vi "stop.vi"(8 "error in (no error)":errorcluster, 10 "stop?":bool, 11 "AtomChipHWC in":refnum<class "AtomChipHWC.lvclass">) -> (0 "error out":errorcluster, 2 "stopped":bool, 3 "AtomChipHWC out":refnum<class "AtomChipHWC.lvclass">)   [LabVIEW 2011, in "Hardware.lvlib" / "HWControllers.lvlib" / "AtomChipHWC.lvclass"]
doc: "Stop current run if input is true, otherwise ask hardware if its finished."
uses:
  AtomChipHWC.lvclass
  AtomChipHWC.lvclass/AtomChipHWC.ctl
  Channels/Digital/DigitalOutput.lvclass
  Channels/VoltOutput/AnalogOutput.lvclass
  Channels/DDSOutput/Generic/DDSOutput.lvclass
  Network Controllers/NetworkCamera/NetworkCamera.lvclass
  IntegrationManagement/CameraManager.lvclass
  HWController.lvclass
  Network Controllers/CameraNetworkController/CameraNetworkController.lvclass
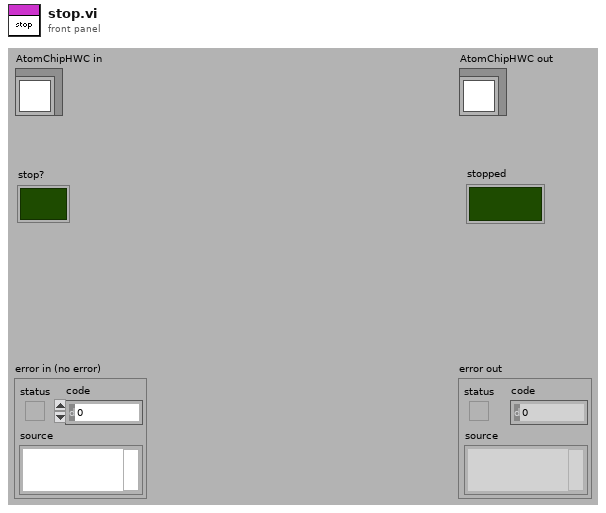
[diagram p1: front panel]
types:
  T1 = enum16{"Ready", "Compiling", "Configured", "Running", "Stopping", "Unresolved Error"}
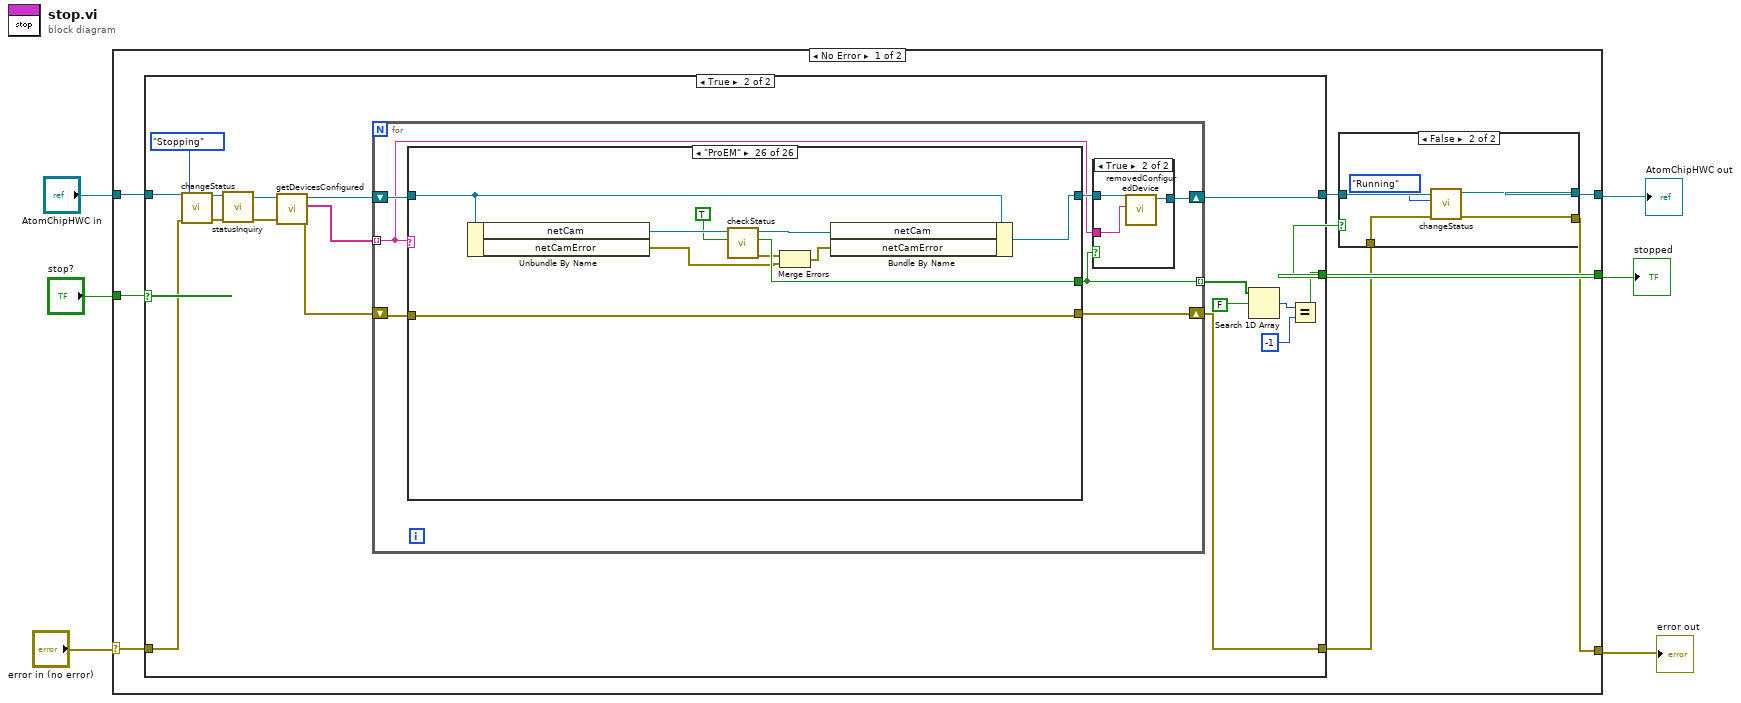
[diagram p0: block diagram]
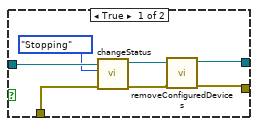
[diagram p2: hidden frame]
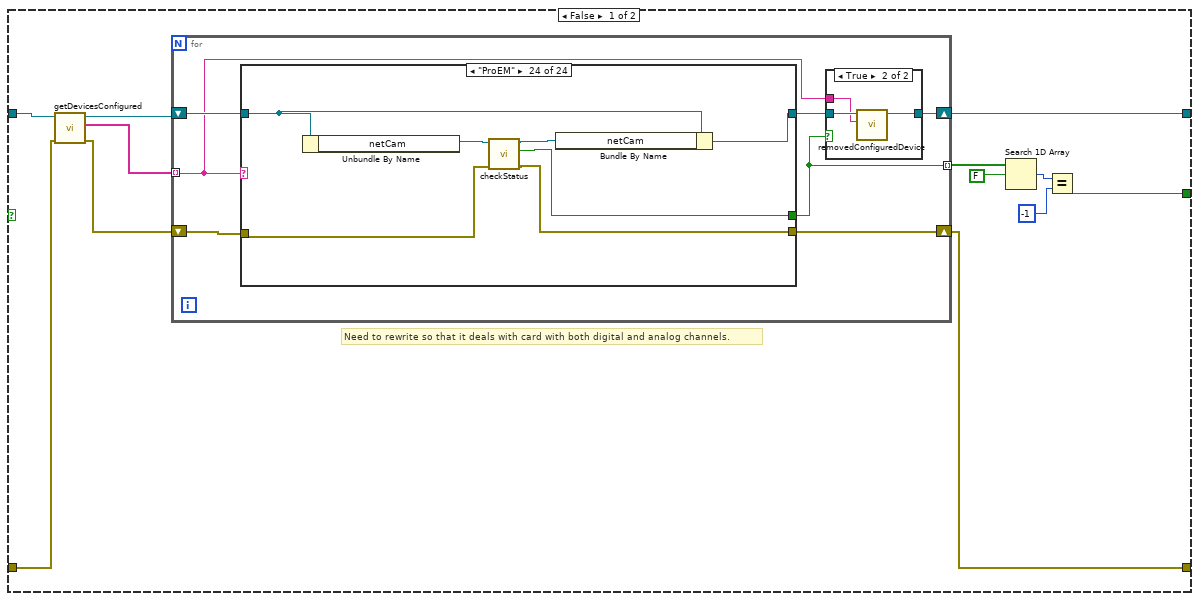
[diagram p3: hidden frame]
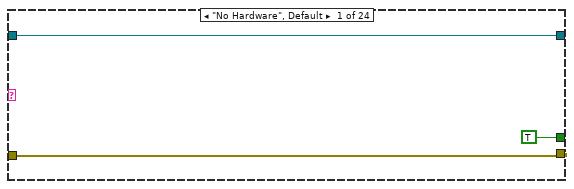
[diagram p5: hidden frame]
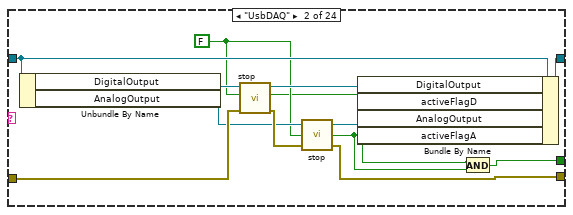
[diagram p6: hidden frame]
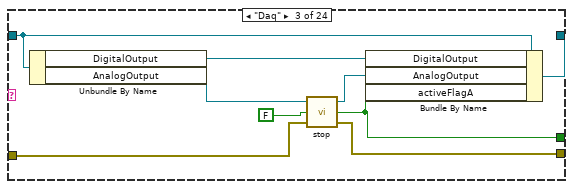
[diagram p7: hidden frame]
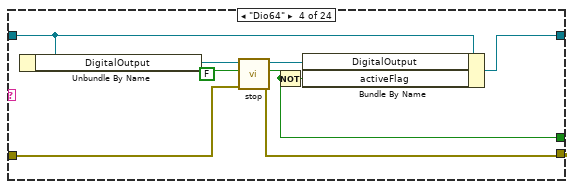
[diagram p8: hidden frame]
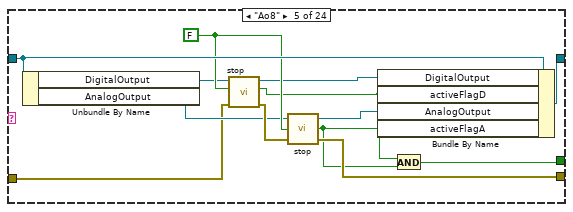
[diagram p9: hidden frame]
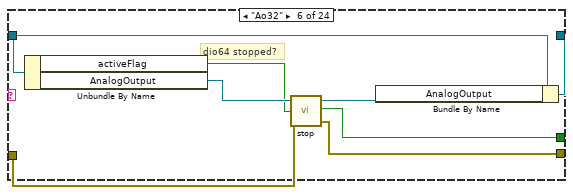
[diagram p10: hidden frame]
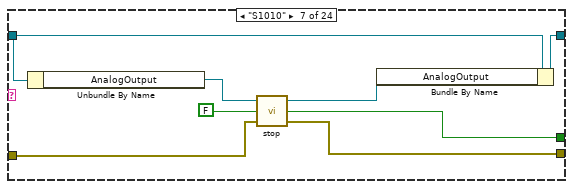
[diagram p11: hidden frame]
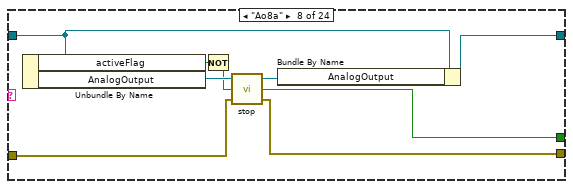
[diagram p12: hidden frame]
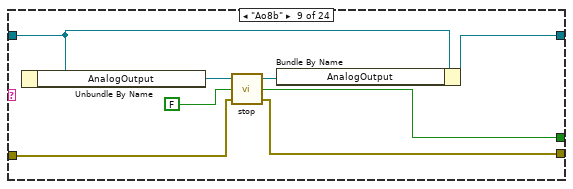
[diagram p13: hidden frame]
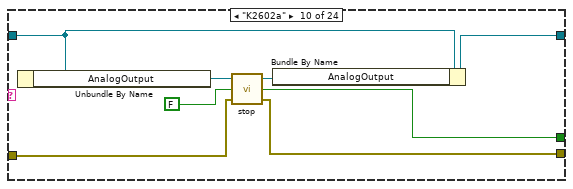
[diagram p14: hidden frame]
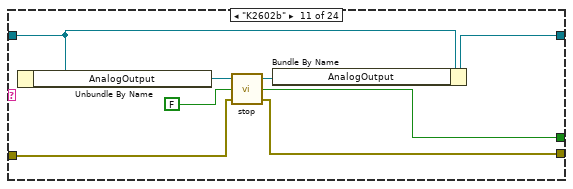
[diagram p15: hidden frame]
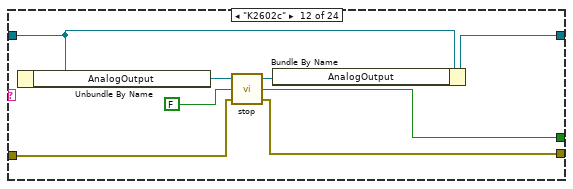
[diagram p16: hidden frame]
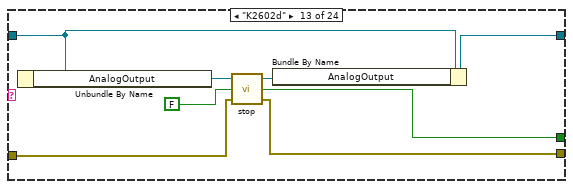
[diagram p17: hidden frame]
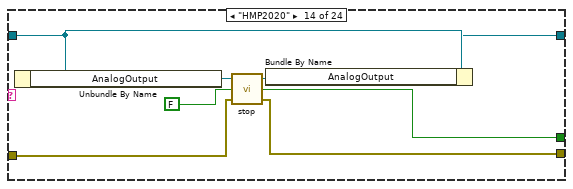
[diagram p18: hidden frame]
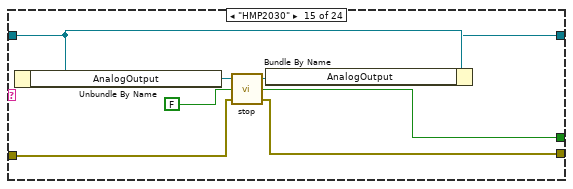
[diagram p19: hidden frame]
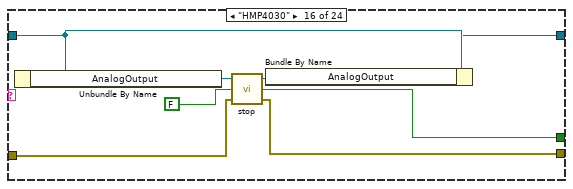
[diagram p20: hidden frame]
diagram:
  n1 = case shown="No Error" "error in (no error)" {
    selector: "error in (no error)" -> [w13 w549]
    tunnel: "AtomChipHWC in" -> [w14 w550]
    tunnel: [w8 w550] -> w5
    tunnel: [w7 w549] -> w3
    tunnel: "stop?" -> [w12 _]
    tunnel: [w9 _] -> w1
    frame No Error {
      n2 = case shown="True" w12 {
        tunnel: w14 -> [w31 w263]
        tunnel: [w38 w261] -> w11
        tunnel: w13 -> [w29 w262]
        tunnel: [w37 w260] -> w10
        tunnel: [w32 w247] -> w9
        frame False {
          # "Need to rewrite so that it deals with card with both digital and analog channels."
          n3 = call "getDevicesConfigured.vi"("error in (no error)"=w29, "HWController.lvclass in"=w31) -> ("error out"=w28:errorcluster, "devicesConfigured"=w27:string[], "HWController.lvclass out"=w30:refnum<class "AtomChipHWC.lvclass">)  [unwired: 7 in]
          n4 = for {
            shift-right: [w40] -> w38
            shift-left: w30 -> [w45]
            tunnel: w27 -> [w41] mode=indexing
            shift-right: [w44] -> w37
            shift-left: w28 -> [w43]
            tunnel: [w42] -> w36 mode=indexing
            n5 = case shown="\"ProEM\"" w41 {
              tunnel: [w52 w64 w74 w79 w95 w104 w112 w115 w123 w131 w139 w147 w155 w163 w171 w179 w186 w194 w203 w212 w222 w231 w238 w245] -> w39
              tunnel: [w51 w61 w69 w81 w88 w101 w109 w119 w127 w135 w143 w151 w159 w167 w175 w183 w190 w198 w207 w216 w220 w227 w234 w241] -> w44
              tunnel: w45 -> [w52 w65 w72 w78 w96 w103 w111 w117 w125 w133 w141 w149 w157 w165 w173 w181 w188 w196 w205 w214 w223 w232 w239 w246]
              tunnel: w43 -> [w51 w59 w66 w82 w89 w99 w107 w120 w128 w136 w144 w152 w160 w168 w176 w184 w191 w199 w208 w217 w224 w228 w235 w242]
              tunnel: [TRUE w53 w67 w76 w84 w98 w105 w118 w126 w134 w142 w150 w158 w166 w174 w182 w189 w197 w206 w215 w221 w226 w233 w240] -> w42
              frame "No Hardware", Default {
              }
              frame "UsbDAQ" {
                w57 = FALSE
                n6 = Unbundle By Name(w65) -> ("DigitalOutput"=w63:refnum<class "DigitalOutput.lvclass">, "AnalogOutput"=w58:refnum<class "AnalogOutput.lvclass">)
                n7 = call-dynamic "stop.vi"("error in (no error)"=w59, "stop"=w57, "DigitalOutput in"=w63) -> ("error out"=w60:errorcluster, "stopped"=w54:bool, "DigitalOutput out"=w62:refnum<class "DigitalOutput.lvclass">)  [unwired: 6 in]
                n8 = call-dynamic "stop.vi"("error in (no error)"=w60, "stop"=w57, "AnalogOutput in"=w58) -> ("error out"=w61:errorcluster, "Stopped"=w55:bool, "AnalogOutput out"=w56:refnum<class "AnalogOutput.lvclass">)
                n9 = Bundle By Name(cluster=w65, "DigitalOutput"=w62, "activeFlagD"=w54, "AnalogOutput"=w56, "activeFlagA"=w55) -> (w64:refnum<class "AtomChipHWC.lvclass">)
                n10 = And(x=w54, y=w55) -> (x .and. y?=w53:bool)
              }
              frame "Daq" {
                n11 = Unbundle By Name(w72) -> ("DigitalOutput"=w68:refnum<class "DigitalOutput.lvclass">, "AnalogOutput"=w71:refnum<class "AnalogOutput.lvclass">)
                n12 = call-dynamic "stop.vi"("error in (no error)"=w66, "stop"=FALSE, "AnalogOutput in"=w71) -> ("error out"=w69:errorcluster, "Stopped"=w67:bool, "AnalogOutput out"=w70:refnum<class "AnalogOutput.lvclass">)
                n13 = Bundle By Name(cluster=w72, "DigitalOutput"=w68, "AnalogOutput"=w70, "activeFlagA"=w67) -> (w74:refnum<class "AtomChipHWC.lvclass">)
              }
              frame "Dio64" {
                n14 = Unbundle By Name(w78) -> ("DigitalOutput"=w83:refnum<class "DigitalOutput.lvclass">)
                n15 = call-dynamic "stop.vi"("error in (no error)"=w82, "stop"=FALSE, "DigitalOutput in"=w83) -> ("error out"=w81:errorcluster, "stopped"=w76:bool, "DigitalOutput out"=w80:refnum<class "DigitalOutput.lvclass">)  [unwired: 6 in]
                n16 = Not(x=w76) -> (.not. x?=w75:bool)
                n17 = Bundle By Name(cluster=w78, "DigitalOutput"=w80, "activeFlag"=w75) -> (w79:refnum<class "AtomChipHWC.lvclass">)
              }
              frame "Ao8" {
                w93 = FALSE
                n18 = Unbundle By Name(w96) -> ("DigitalOutput"=w92:refnum<class "DigitalOutput.lvclass">, "AnalogOutput"=w91:refnum<class "AnalogOutput.lvclass">)
                n19 = call-dynamic "stop.vi"("error in (no error)"=w89, "stop"=w93, "DigitalOutput in"=w92) -> ("error out"=w94:errorcluster, "stopped"=w86:bool, "DigitalOutput out"=w90:refnum<class "DigitalOutput.lvclass">)  [unwired: 6 in]
                n20 = call-dynamic "stop.vi"("error in (no error)"=w94, "stop"=w93, "AnalogOutput in"=w91) -> ("error out"=w88:errorcluster, "Stopped"=w85:bool, "AnalogOutput out"=w87:refnum<class "AnalogOutput.lvclass">)
                n21 = Bundle By Name(cluster=w96, "DigitalOutput"=w90, "activeFlagD"=w86, "AnalogOutput"=w87, "activeFlagA"=w85) -> (w95:refnum<class "AtomChipHWC.lvclass">)
                n22 = And(x=w86, y=w85) -> (x .and. y?=w84:bool)
              }
              frame "Ao32" {
                # "dio64 stopped?"
                n23 = Unbundle By Name(w103) -> ("activeFlag"=w97:bool, "AnalogOutput"=w102:refnum<class "AnalogOutput.lvclass">)
                n24 = call-dynamic "stop.vi"("error in (no error)"=w99, "stop"=w97, "AnalogOutput in"=w102) -> ("error out"=w101:errorcluster, "Stopped"=w98:bool, "AnalogOutput out"=w100:refnum<class "AnalogOutput.lvclass">)
                n25 = Bundle By Name(cluster=w103, "AnalogOutput"=w100) -> (w104:refnum<class "AtomChipHWC.lvclass">)
              }
              frame "S1010" {
                n26 = Unbundle By Name(w111) -> ("AnalogOutput"=w110:refnum<class "AnalogOutput.lvclass">)
                n27 = call-dynamic "stop.vi"("error in (no error)"=w107, "stop"=FALSE, "AnalogOutput in"=w110) -> ("error out"=w109:errorcluster, "Stopped"=w105:bool, "AnalogOutput out"=w108:refnum<class "AnalogOutput.lvclass">)
                n28 = Bundle By Name(cluster=w111, "AnalogOutput"=w108) -> (w112:refnum<class "AtomChipHWC.lvclass">)
              }
              frame "Ao8a" {
                n29 = Unbundle By Name(w117) -> ("activeFlag"=w114:bool, "AnalogOutput"=w121:refnum<class "AnalogOutput.lvclass">)
                n30 = Not(x=w114) -> (.not. x?=w113:bool)
                n31 = call-dynamic "stop.vi"("error in (no error)"=w120, "stop"=w113, "AnalogOutput in"=w121) -> ("error out"=w119:errorcluster, "Stopped"=w118:bool, "AnalogOutput out"=w116:refnum<class "AnalogOutput.lvclass">)
                n32 = Bundle By Name(cluster=w117, "AnalogOutput"=w116) -> (w115:refnum<class "AtomChipHWC.lvclass">)
              }
              frame "Ao8b" {
                n33 = Unbundle By Name(w125) -> ("AnalogOutput"=w129:refnum<class "AnalogOutput.lvclass">)
                n34 = call-dynamic "stop.vi"("error in (no error)"=w128, "stop"=FALSE, "AnalogOutput in"=w129) -> ("error out"=w127:errorcluster, "Stopped"=w126:bool, "AnalogOutput out"=w124:refnum<class "AnalogOutput.lvclass">)
                n35 = Bundle By Name(cluster=w125, "AnalogOutput"=w124) -> (w123:refnum<class "AtomChipHWC.lvclass">)
              }
              frame "K2602a" {
                n36 = Unbundle By Name(w133) -> ("AnalogOutput"=w137:refnum<class "AnalogOutput.lvclass">)
                n37 = call-dynamic "stop.vi"("error in (no error)"=w136, "stop"=FALSE, "AnalogOutput in"=w137) -> ("error out"=w135:errorcluster, "Stopped"=w134:bool, "AnalogOutput out"=w132:refnum<class "AnalogOutput.lvclass">)
                n38 = Bundle By Name(cluster=w133, "AnalogOutput"=w132) -> (w131:refnum<class "AtomChipHWC.lvclass">)
              }
              frame "K2602b" {
                n39 = Unbundle By Name(w141) -> ("AnalogOutput"=w145:refnum<class "AnalogOutput.lvclass">)
                n40 = call-dynamic "stop.vi"("error in (no error)"=w144, "stop"=FALSE, "AnalogOutput in"=w145) -> ("error out"=w143:errorcluster, "Stopped"=w142:bool, "AnalogOutput out"=w140:refnum<class "AnalogOutput.lvclass">)
                n41 = Bundle By Name(cluster=w141, "AnalogOutput"=w140) -> (w139:refnum<class "AtomChipHWC.lvclass">)
              }
              frame "K2602c" {
                n42 = Unbundle By Name(w149) -> ("AnalogOutput"=w153:refnum<class "AnalogOutput.lvclass">)
                n43 = call-dynamic "stop.vi"("error in (no error)"=w152, "stop"=FALSE, "AnalogOutput in"=w153) -> ("error out"=w151:errorcluster, "Stopped"=w150:bool, "AnalogOutput out"=w148:refnum<class "AnalogOutput.lvclass">)
                n44 = Bundle By Name(cluster=w149, "AnalogOutput"=w148) -> (w147:refnum<class "AtomChipHWC.lvclass">)
              }
              frame "K2602d" {
                n45 = Unbundle By Name(w157) -> ("AnalogOutput"=w161:refnum<class "AnalogOutput.lvclass">)
                n46 = call-dynamic "stop.vi"("error in (no error)"=w160, "stop"=FALSE, "AnalogOutput in"=w161) -> ("error out"=w159:errorcluster, "Stopped"=w158:bool, "AnalogOutput out"=w156:refnum<class "AnalogOutput.lvclass">)
                n47 = Bundle By Name(cluster=w157, "AnalogOutput"=w156) -> (w155:refnum<class "AtomChipHWC.lvclass">)
              }
              frame "HMP2020" {
                n48 = Unbundle By Name(w165) -> ("AnalogOutput"=w169:refnum<class "AnalogOutput.lvclass">)
                n49 = call-dynamic "stop.vi"("error in (no error)"=w168, "stop"=FALSE, "AnalogOutput in"=w169) -> ("error out"=w167:errorcluster, "Stopped"=w166:bool, "AnalogOutput out"=w164:refnum<class "AnalogOutput.lvclass">)
                n50 = Bundle By Name(cluster=w165, "AnalogOutput"=w164) -> (w163:refnum<class "AtomChipHWC.lvclass">)
              }
              frame "HMP2030" {
                n51 = Unbundle By Name(w173) -> ("AnalogOutput"=w177:refnum<class "AnalogOutput.lvclass">)
                n52 = call-dynamic "stop.vi"("error in (no error)"=w176, "stop"=FALSE, "AnalogOutput in"=w177) -> ("error out"=w175:errorcluster, "Stopped"=w174:bool, "AnalogOutput out"=w172:refnum<class "AnalogOutput.lvclass">)
                n53 = Bundle By Name(cluster=w173, "AnalogOutput"=w172) -> (w171:refnum<class "AtomChipHWC.lvclass">)
              }
              frame "HMP4030" {
                n54 = Unbundle By Name(w181) -> ("AnalogOutput"=w185:refnum<class "AnalogOutput.lvclass">)
                n55 = call-dynamic "stop.vi"("error in (no error)"=w184, "stop"=FALSE, "AnalogOutput in"=w185) -> ("error out"=w183:errorcluster, "Stopped"=w182:bool, "AnalogOutput out"=w180:refnum<class "AnalogOutput.lvclass">)
                n56 = Bundle By Name(cluster=w181, "AnalogOutput"=w180) -> (w179:refnum<class "AtomChipHWC.lvclass">)
              }
              frame "SpinCoreDDS0" {
                n57 = Unbundle By Name(w188) -> ("DDSOutput"=w192:refnum<class "DDSOutput.lvclass">)
                n58 = call-dynamic "stop.vi"("error in (no error)"=w191, "DDSOutput in"=w192) -> ("error out"=w190:errorcluster, "hasStopped"=w189:bool, "DDSOutput out"=w187:refnum<class "DDSOutput.lvclass">)  [unwired: 7 in]
                n59 = Bundle By Name(cluster=w188, "DDSOutput"=w187) -> (w186:refnum<class "AtomChipHWC.lvclass">)
              }
              frame "SpinCoreDDS1" {
                n60 = Unbundle By Name(w196) -> ("DDSOutput"=w200:refnum<class "DDSOutput.lvclass">)
                n61 = call-dynamic "stop.vi"("error in (no error)"=w199, "stop?"=FALSE, "DDSOutput in"=w200) -> ("error out"=w198:errorcluster, "hasStopped"=w197:bool, "DDSOutput out"=w195:refnum<class "DDSOutput.lvclass">)  [unwired: 6 in]
                n62 = Bundle By Name(cluster=w196, "DDSOutput"=w195) -> (w194:refnum<class "AtomChipHWC.lvclass">)
              }
              frame "k3390" {
                # "stop when Dio64 has stopped."
                n63 = Unbundle By Name(w205) -> ("DDSOutput"=w209:refnum<class "DDSOutput.lvclass">, "activeFlag"=w201:bool)
                n64 = Not(x=w201) -> (.not. x?=w202:bool)
                n65 = call-dynamic "stop.vi"("error in (no error)"=w208, "stop?"=w202, "DDSOutput in"=w209) -> ("error out"=w207:errorcluster, "hasStopped"=w206:bool, "DDSOutput out"=w204:refnum<class "DDSOutput.lvclass">)  [unwired: 6 in]
                n66 = Bundle By Name(cluster=w205, "DDSOutput"=w204) -> (w203:refnum<class "AtomChipHWC.lvclass">)
              }
              frame "CQTDDS0" {
                # "stop when Dio64 has stopped."
                n67 = Unbundle By Name(w214) -> ("DDSOutput"=w218:refnum<class "DDSOutput.lvclass">, "activeFlag"=w211:bool)
                n68 = Not(x=w211) -> (.not. x?=w210:bool)
                n69 = call-dynamic "stop.vi"("error in (no error)"=w217, "stop?"=w210, "DDSOutput in"=w218) -> ("error out"=w216:errorcluster, "hasStopped"=w215:bool, "DDSOutput out"=w213:refnum<class "DDSOutput.lvclass">)  [unwired: 6 in]
                n70 = Bundle By Name(cluster=w214, "DDSOutput"=w213) -> (w212:refnum<class "AtomChipHWC.lvclass">)
              }
              frame "oldPixelfly", "oldProEM_WinX32" {
                n71 = Unbundle By Name(w223) -> ("CameraNetworkController"=w225:refnum<class "CameraNetworkController.lvclass">)
                n72 = call "stop.vi"("error in (no error)"=w224, "CameraNetworkController in"=w225) -> ("error out"=w220:errorcluster, "stopped?"=w221:bool, "CameraNetworkController out"=w219:refnum<class "CameraNetworkController.lvclass">)  [unwired: 7 in]
                n73 = Bundle By Name(cluster=w223, "CameraNetworkController"=w219) -> (w222:refnum<class "AtomChipHWC.lvclass">)
              }
              frame "Pixelfly" {
                n74 = Unbundle By Name(w232) -> ("netCam"=w230:refnum<class "NetworkCamera.lvclass">)
                n75 = call-dynamic "checkStatus.vi"("error in (no error)"=w228, "NetworkCamera in"=w230) -> ("error out"=w227:errorcluster, "stopped?"=w226:bool, "NetworkCamera out"=w229:refnum<class "NetworkCamera.lvclass">)  [unwired: 7 in]
                n76 = Bundle By Name(cluster=w232, "netCam"=w229) -> (w231:refnum<class "AtomChipHWC.lvclass">)
              }
              frame "Pixis" {
                n77 = Unbundle By Name(w239) -> ("netCam"=w237:refnum<class "NetworkCamera.lvclass">)
                n78 = call-dynamic "checkStatus.vi"("error in (no error)"=w235, "NetworkCamera in"=w237) -> ("error out"=w234:errorcluster, "stopped?"=w233:bool, "NetworkCamera out"=w236:refnum<class "NetworkCamera.lvclass">)  [unwired: 7 in]
                n79 = Bundle By Name(cluster=w239, "netCam"=w236) -> (w238:refnum<class "AtomChipHWC.lvclass">)
              }
              frame "ProEM" {
                n80 = Unbundle By Name(w246) -> ("netCam"=w244:refnum<class "NetworkCamera.lvclass">)
                n81 = call-dynamic "checkStatus.vi"("error in (no error)"=w242, "NetworkCamera in"=w244) -> ("error out"=w241:errorcluster, "stopped?"=w240:bool, "NetworkCamera out"=w243:refnum<class "NetworkCamera.lvclass">)  [unwired: 7 in]
                n82 = Bundle By Name(cluster=w246, "netCam"=w243) -> (w245:refnum<class "AtomChipHWC.lvclass">)
              }
            }
            n83 = case shown="True" w42 {
              tunnel: w41 -> [_ w47]
              tunnel: [w46 w48] -> w40
              tunnel: w39 -> [w46 w49]
              frame False {
              }
              frame True {
                n84 = call-dynamic "removedConfiguredDevice.vi"("device"=w47, "HWController in"=w49) -> ("HWController out"=w48:refnum<class "AtomChipHWC.lvclass">)  [unwired: 8 in, 1 out]
              }
            }
          }
          n85 = Search 1D Array(1D array=w36, element=FALSE) -> (index of element=w34:i32)  [unwired: 1 in]
          n86 = Equal?(x=w34, y=-1) -> (x = y?=w32:bool)
        }
        frame True {
          n87 = call "changeStatus.vi"("error in (no error)"=w262, "status"=T1."Stopping", "HWController in"=w263) -> ("error out"=w258:errorcluster, "HWController out"=w259:refnum<class "AtomChipHWC.lvclass">)  [unwired: 7 in]
          n88 = call-dynamic "statusInquiry.vi"("error in (no error)"=w258, "HWController in"=w259) -> ("error out"=w254:errorcluster, "HWController out"=w257:refnum<class "AtomChipHWC.lvclass">)  [unwired: 8 in]
          n89 = call "getDevicesConfigured.vi"("error in (no error)"=w254, "HWController.lvclass in"=w257) -> ("error out"=w253:errorcluster, "devicesConfigured"=w255:string[], "HWController.lvclass out"=w256:refnum<class "AtomChipHWC.lvclass">)  [unwired: 7 in]
          n90 = for {
            tunnel: w255 -> [w265] mode=indexing
            shift-right: [w266] -> w261
            shift-left: w256 -> [w270]
            shift-right: [w268] -> w260
            shift-left: w253 -> [w269]
            tunnel: [w264] -> w248 mode=indexing
            n91 = case shown="\"ProEM\"" w265 {
              tunnel: [w277 w284 w317 w325 w342 w369 w375 w383 w391 w399 w408 w417 w426 w435 w444 w453 w462 w471 w482 w491 w500 w509 w519 w528 w537 w547] -> w267
              tunnel: [w276 w278 w310 w320 w329 w361 w370 w381 w387 w395 w404 w413 w422 w431 w440 w449 w458 w467 w476 w485 w494 w503 w514 w527 w536 w546] -> w268
              tunnel: w270 -> [w277 w283 w316 w326 w341 w368 w376 w385 w393 w400 w409 w418 w427 w436 w445 w454 w463 w472 w483 w492 w501 w510 w520 w529 w538 w548]
              tunnel: w269 -> [w276 w278 w310 w320 w329 w361 w370 w381 w387 w395 w404 w413 w422 w431 w440 w449 w458 w467 w476 w485 w494 w503 w514 w527 w536 w546]
              tunnel: [FALSE w282 w313 w324 w334 w364 w374 TRUE TRUE w398 w407 w416 w425 w434 w443 w452 w461 w470 w480 w489 w498 w507 w515 w521 w530 w542] -> w264
              frame "No Hardware", Default {
              }
              frame "UsbDAQ" {
                n92 = Unbundle By Name(w283) -> ("DigitalOutput"=w291:refnum<class "DigitalOutput.lvclass">, "AnalogOutput"=w288:refnum<class "AnalogOutput.lvclass">, "activeFlagD"=w290:bool, "activeFlagA"=w287:bool, "UsbDAQError"=w279:errorcluster)
                n93 = case shown="False" w290 {
                  selector: w290 -> [_ w307]
                  tunnel: w291 -> [w306 w309]
                  tunnel: [w305 w309] -> w289
                  tunnel: w279 -> [w304 w308]
                  tunnel: [w303 w308] -> w281
                  tunnel: [w301 w307] -> w286
                  frame False {
                    n94 = call-dynamic "stop.vi"("error in (no error)"=w304, "stop"=TRUE, "DigitalOutput in"=w306) -> ("error out"=w303:errorcluster, "stopped"=w301:bool, "DigitalOutput out"=w305:refnum<class "DigitalOutput.lvclass">)  [unwired: 6 in]
                  }
                  frame True {
                  }
                }
                n95 = case shown="False" w287 {
                  selector: w287 -> [_ w298]
                  tunnel: w281 -> [w297 w299]
                  tunnel: w288 -> [w296 w300]
                  tunnel: [w294 w300] -> w285
                  tunnel: [w293 w299] -> w280
                  tunnel: [w292 w298] -> w282
                  frame False {
                    n96 = call-dynamic "stop.vi"("error in (no error)"=w297, "stop"=TRUE, "AnalogOutput in"=w296) -> ("error out"=w293:errorcluster, "Stopped"=w292:bool, "AnalogOutput out"=w294:refnum<class "AnalogOutput.lvclass">)
                  }
                  frame True {
                  }
                }
                n97 = Bundle By Name(cluster=w283, "DigitalOutput"=w289, "AnalogOutput"=w285, "activeFlagD"=w286, "activeFlagA"=w282, "UsbDAQError"=w280) -> (w284:refnum<class "AtomChipHWC.lvclass">)
              }
              frame "Daq" {
                n98 = Unbundle By Name(w316) -> ("DigitalOutput"=w315:refnum<class "DigitalOutput.lvclass">, "AnalogOutput"=w319:refnum<class "AnalogOutput.lvclass">, "daqError"=w311:errorcluster)
                n99 = call-dynamic "stop.vi"("error in (no error)"=w311, "stop"=TRUE, "AnalogOutput in"=w319) -> ("error out"=w312:errorcluster, "Stopped"=w313:bool, "AnalogOutput out"=w318:refnum<class "AnalogOutput.lvclass">)
                n100 = Bundle By Name(cluster=w316, "DigitalOutput"=w315, "AnalogOutput"=w318, "activeFlagA"=w313, "daqError"=w312) -> (w317:refnum<class "AtomChipHWC.lvclass">)
              }
              frame "Dio64" {
                n101 = Unbundle By Name(w326) -> ("DigitalOutput"=w328:refnum<class "DigitalOutput.lvclass">, "Dio64Error"=w321:errorcluster)
                n102 = call-dynamic "stop.vi"("error in (no error)"=w321, "stop"=TRUE, "DigitalOutput in"=w328) -> ("error out"=w322:errorcluster, "stopped"=w324:bool, "DigitalOutput out"=w327:refnum<class "DigitalOutput.lvclass">)  [unwired: 6 in]
                n103 = Bundle By Name(cluster=w326, "DigitalOutput"=w327, "activeFlag"=w324, "Dio64Error"=w322) -> (w325:refnum<class "AtomChipHWC.lvclass">)
              }
              frame "Ao8" {
                n104 = Unbundle By Name(w341) -> ("DigitalOutput"=w340:refnum<class "DigitalOutput.lvclass">, "AnalogOutput"=w331:refnum<class "AnalogOutput.lvclass">, "activeFlagD"=w339:bool, "activeFlagA"=w333:bool, "Ao8Error"=w330:errorcluster)
                n105 = case shown="False" w339 {
                  selector: w339 -> [_ w358]
                  tunnel: w340 -> [w357 w360]
                  tunnel: [w356 w360] -> w338
                  tunnel: w330 -> [w355 w359]
                  tunnel: [w354 w359] -> w337
                  tunnel: [w352 w358] -> w336
                  frame False {
                    n106 = call-dynamic "stop.vi"("error in (no error)"=w355, "stop"=TRUE, "DigitalOutput in"=w357) -> ("error out"=w354:errorcluster, "stopped"=w352:bool, "DigitalOutput out"=w356:refnum<class "DigitalOutput.lvclass">)  [unwired: 6 in]
                  }
                  frame True {
                  }
                }
                n107 = case shown="False" w333 {
                  selector: w333 -> [_ w349]
                  tunnel: w337 -> [w348 w350]
                  tunnel: w331 -> [w347 w351]
                  tunnel: [w345 w351] -> w335
                  tunnel: [w344 w350] -> w332
                  tunnel: [w343 w349] -> w334
                  frame False {
                    n108 = call-dynamic "stop.vi"("error in (no error)"=w348, "stop"=TRUE, "AnalogOutput in"=w347) -> ("error out"=w344:errorcluster, "Stopped"=w343:bool, "AnalogOutput out"=w345:refnum<class "AnalogOutput.lvclass">)
                  }
                  frame True {
                  }
                }
                n109 = Bundle By Name(cluster=w341, "DigitalOutput"=w338, "AnalogOutput"=w335, "activeFlagD"=w336, "activeFlagA"=w334, "Ao8Error"=w332) -> (w342:refnum<class "AtomChipHWC.lvclass">)
              }
              frame "Ao32" {
                n110 = Unbundle By Name(w368) -> ("AnalogOutput"=w367:refnum<class "AnalogOutput.lvclass">, "Ao32Error"=w363:errorcluster)
                n111 = call-dynamic "stop.vi"("error in (no error)"=w363, "stop"=TRUE, "AnalogOutput in"=w367) -> ("error out"=w362:errorcluster, "Stopped"=w364:bool, "AnalogOutput out"=w366:refnum<class "AnalogOutput.lvclass">)
                n112 = Bundle By Name(cluster=w368, "AnalogOutput"=w366, "Ao32Error"=w362) -> (w369:refnum<class "AtomChipHWC.lvclass">)
              }
              frame "S1010" {
                n113 = Unbundle By Name(w376) -> ("AnalogOutput"=w378:refnum<class "AnalogOutput.lvclass">, "daqError"=w372:errorcluster)
                n114 = call-dynamic "stop.vi"("error in (no error)"=w372, "stop"=TRUE, "AnalogOutput in"=w378) -> ("error out"=w371:errorcluster, "Stopped"=w374:bool, "AnalogOutput out"=w377:refnum<class "AnalogOutput.lvclass">)
                n115 = Bundle By Name(cluster=w376, "AnalogOutput"=w377, "daqError"=w371) -> (w375:refnum<class "AtomChipHWC.lvclass">)
              }
              frame "ICCamera" {
                n116 = Unbundle By Name(w385) -> ("CameraManager"=w386:refnum<class "CameraManager.lvclass">, "ICCameraError"=w380:errorcluster)
                n117 = call-dynamic "stopSnapping.vi"("error in (no error)"=w380, "CameraManager in"=w386) -> ("error out"=w379:errorcluster, "CameraManager out"=w384:refnum<class "CameraManager.lvclass">)  [unwired: 8 in]
                n118 = Bundle By Name(cluster=w385, "CameraManager"=w384, "ICCameraError"=w379) -> (w383:refnum<class "AtomChipHWC.lvclass">)
              }
              frame "AndorIKon" {
                n119 = Unbundle By Name(w393) -> ("CameraManager"=w394:refnum<class "CameraManager.lvclass">, "AndorIkonError"=w389:errorcluster)
                n120 = call-dynamic "stopSnapping.vi"("error in (no error)"=w389, "CameraManager in"=w394) -> ("error out"=w388:errorcluster, "CameraManager out"=w392:refnum<class "CameraManager.lvclass">)  [unwired: 8 in]
                n121 = Bundle By Name(cluster=w393, "CameraManager"=w392, "AndorIkonError"=w388) -> (w391:refnum<class "AtomChipHWC.lvclass">)
              }
              frame "Ao8a" {
                n122 = Unbundle By Name(w400) -> ("AnalogOutput"=w402:refnum<class "AnalogOutput.lvclass">, "Ao8aError"=w397:errorcluster)
                n123 = call-dynamic "stop.vi"("error in (no error)"=w397, "stop"=TRUE, "AnalogOutput in"=w402) -> ("error out"=w396:errorcluster, "Stopped"=w398:bool, "AnalogOutput out"=w401:refnum<class "AnalogOutput.lvclass">)
                n124 = Bundle By Name(cluster=w400, "AnalogOutput"=w401, "Ao8aError"=w396) -> (w399:refnum<class "AtomChipHWC.lvclass">)
              }
              frame "Ao8b" {
                n125 = Unbundle By Name(w409) -> ("AnalogOutput"=w411:refnum<class "AnalogOutput.lvclass">, "Ao8bError"=w406:errorcluster)
                n126 = call-dynamic "stop.vi"("error in (no error)"=w406, "stop"=TRUE, "AnalogOutput in"=w411) -> ("error out"=w405:errorcluster, "Stopped"=w407:bool, "AnalogOutput out"=w410:refnum<class "AnalogOutput.lvclass">)
                n127 = Bundle By Name(cluster=w409, "AnalogOutput"=w410, "Ao8bError"=w405) -> (w408:refnum<class "AtomChipHWC.lvclass">)
              }
              frame "K2602a" {
                n128 = Unbundle By Name(w418) -> ("AnalogOutput"=w420:refnum<class "AnalogOutput.lvclass">, "K2602aError"=w415:errorcluster)
                n129 = call-dynamic "stop.vi"("error in (no error)"=w415, "stop"=TRUE, "AnalogOutput in"=w420) -> ("error out"=w414:errorcluster, "Stopped"=w416:bool, "AnalogOutput out"=w419:refnum<class "AnalogOutput.lvclass">)
                n130 = Bundle By Name(cluster=w418, "AnalogOutput"=w419, "K2602aError"=w414) -> (w417:refnum<class "AtomChipHWC.lvclass">)
              }
              frame "K2602b" {
                n131 = Unbundle By Name(w427) -> ("AnalogOutput"=w429:refnum<class "AnalogOutput.lvclass">, "K2602bError"=w424:errorcluster)
                n132 = call-dynamic "stop.vi"("error in (no error)"=w424, "stop"=TRUE, "AnalogOutput in"=w429) -> ("error out"=w423:errorcluster, "Stopped"=w425:bool, "AnalogOutput out"=w428:refnum<class "AnalogOutput.lvclass">)
                n133 = Bundle By Name(cluster=w427, "AnalogOutput"=w428, "K2602bError"=w423) -> (w426:refnum<class "AtomChipHWC.lvclass">)
              }
              frame "K2602c" {
                n134 = Unbundle By Name(w436) -> ("AnalogOutput"=w438:refnum<class "AnalogOutput.lvclass">, "K2602cError"=w433:errorcluster)
                n135 = call-dynamic "stop.vi"("error in (no error)"=w433, "stop"=TRUE, "AnalogOutput in"=w438) -> ("error out"=w432:errorcluster, "Stopped"=w434:bool, "AnalogOutput out"=w437:refnum<class "AnalogOutput.lvclass">)
                n136 = Bundle By Name(cluster=w436, "AnalogOutput"=w437, "K2602cError"=w432) -> (w435:refnum<class "AtomChipHWC.lvclass">)
              }
              frame "K2602d" {
                n137 = Unbundle By Name(w445) -> ("AnalogOutput"=w447:refnum<class "AnalogOutput.lvclass">, "K2602dError"=w442:errorcluster)
                n138 = call-dynamic "stop.vi"("error in (no error)"=w442, "stop"=TRUE, "AnalogOutput in"=w447) -> ("error out"=w441:errorcluster, "Stopped"=w443:bool, "AnalogOutput out"=w446:refnum<class "AnalogOutput.lvclass">)
                n139 = Bundle By Name(cluster=w445, "AnalogOutput"=w446, "K2602dError"=w441) -> (w444:refnum<class "AtomChipHWC.lvclass">)
              }
              frame "HMP2020" {
                n140 = Unbundle By Name(w454) -> ("AnalogOutput"=w456:refnum<class "AnalogOutput.lvclass">, "2020Error"=w451:errorcluster)
                n141 = call-dynamic "stop.vi"("error in (no error)"=w451, "stop"=TRUE, "AnalogOutput in"=w456) -> ("error out"=w450:errorcluster, "Stopped"=w452:bool, "AnalogOutput out"=w455:refnum<class "AnalogOutput.lvclass">)
                n142 = Bundle By Name(cluster=w454, "AnalogOutput"=w455, "2020Error"=w450) -> (w453:refnum<class "AtomChipHWC.lvclass">)
              }
              frame "HMP2030" {
                n143 = Unbundle By Name(w463) -> ("AnalogOutput"=w465:refnum<class "AnalogOutput.lvclass">, "2030Error"=w460:errorcluster)
                n144 = call-dynamic "stop.vi"("error in (no error)"=w460, "stop"=TRUE, "AnalogOutput in"=w465) -> ("error out"=w459:errorcluster, "Stopped"=w461:bool, "AnalogOutput out"=w464:refnum<class "AnalogOutput.lvclass">)
                n145 = Bundle By Name(cluster=w463, "AnalogOutput"=w464, "2030Error"=w459) -> (w462:refnum<class "AtomChipHWC.lvclass">)
              }
              frame "HMP4030" {
                n146 = Unbundle By Name(w472) -> ("AnalogOutput"=w474:refnum<class "AnalogOutput.lvclass">, "4030Error"=w469:errorcluster)
                n147 = call-dynamic "stop.vi"("error in (no error)"=w469, "stop"=TRUE, "AnalogOutput in"=w474) -> ("error out"=w468:errorcluster, "Stopped"=w470:bool, "AnalogOutput out"=w473:refnum<class "AnalogOutput.lvclass">)
                n148 = Bundle By Name(cluster=w472, "AnalogOutput"=w473, "4030Error"=w468) -> (w471:refnum<class "AtomChipHWC.lvclass">)
              }
              frame "SpinCoreDDS0" {
                n149 = Unbundle By Name(w483) -> ("DDSOutput"=w484:refnum<class "DDSOutput.lvclass">, "DDS0Error"=w478:errorcluster)
                n150 = call-dynamic "stop.vi"("error in (no error)"=w478, "stop?"=TRUE, "DDSOutput in"=w484) -> ("error out"=w477:errorcluster, "hasStopped"=w480:bool, "DDSOutput out"=w481:refnum<class "DDSOutput.lvclass">)  [unwired: 6 in]
                n151 = Bundle By Name(cluster=w483, "DDSOutput"=w481, "DDS0Error"=w477) -> (w482:refnum<class "AtomChipHWC.lvclass">)
              }
              frame "k3390" {
                n152 = Unbundle By Name(w492) -> ("DDSOutput"=w493:refnum<class "DDSOutput.lvclass">, "DDS1Error"=w487:errorcluster)
                n153 = call-dynamic "stop.vi"("error in (no error)"=w487, "stop?"=TRUE, "DDSOutput in"=w493) -> ("error out"=w486:errorcluster, "hasStopped"=w489:bool, "DDSOutput out"=w490:refnum<class "DDSOutput.lvclass">)  [unwired: 6 in]
                n154 = Bundle By Name(cluster=w492, "DDSOutput"=w490, "DDS1Error"=w486) -> (w491:refnum<class "AtomChipHWC.lvclass">)
              }
              frame "SpinCoreDDS1" {
                n155 = Unbundle By Name(w501) -> ("DDSOutput"=w502:refnum<class "DDSOutput.lvclass">, "DDS1Error"=w495:errorcluster)
                n156 = call-dynamic "stop.vi"("error in (no error)"=w495, "stop?"=TRUE, "DDSOutput in"=w502) -> ("error out"=w496:errorcluster, "hasStopped"=w498:bool, "DDSOutput out"=w499:refnum<class "DDSOutput.lvclass">)  [unwired: 6 in]
                n157 = Bundle By Name(cluster=w501, "DDSOutput"=w499, "DDS1Error"=w496) -> (w500:refnum<class "AtomChipHWC.lvclass">)
              }
              frame "CQTDDS0" {
                n158 = Unbundle By Name(w510) -> ("DDSOutput"=w511:refnum<class "DDSOutput.lvclass">, "DDS0Error"=w504:errorcluster)
                n159 = call-dynamic "stop.vi"("error in (no error)"=w504, "stop?"=TRUE, "DDSOutput in"=w511) -> ("error out"=w505:errorcluster, "hasStopped"=w507:bool, "DDSOutput out"=w508:refnum<class "DDSOutput.lvclass">)  [unwired: 6 in]
                n160 = Bundle By Name(cluster=w510, "DDSOutput"=w508, "DDS0Error"=w505) -> (w509:refnum<class "AtomChipHWC.lvclass">)
              }
              frame "oldPixelfly", "oldProEM_WinX32" {
                n161 = Unbundle By Name(w520) -> ("CameraNetworkController"=w518:refnum<class "CameraNetworkController.lvclass">, "CameraNError"=w513:errorcluster)
                n162 = call "stop.vi"("error in (no error)"=w513, "stop"=TRUE, "CameraNetworkController in"=w518) -> ("error out"=w512:errorcluster, "stopped?"=w515:bool, "CameraNetworkController out"=w517:refnum<class "CameraNetworkController.lvclass">)  [unwired: 6 in]
                n163 = Bundle By Name(cluster=w520, "CameraNetworkController"=w517, "CameraNError"=w512) -> (w519:refnum<class "AtomChipHWC.lvclass">)
              }
              frame "Pixelfly" {
                n164 = Unbundle By Name(w529) -> ("netCam"=w525:refnum<class "NetworkCamera.lvclass">, "netCamError"=w524:errorcluster)
                n165 = call-dynamic "checkStatus.vi"("error in (no error)"=w524, "stop"=TRUE, "NetworkCamera in"=w525) -> ("error out"=w523:errorcluster, "stopped?"=w521:bool, "NetworkCamera out"=w526:refnum<class "NetworkCamera.lvclass">)  [unwired: 6 in]
                n166 = Bundle By Name(cluster=w529, "netCam"=w526, "netCamError"=w523) -> (w528:refnum<class "AtomChipHWC.lvclass">)
              }
              frame "Pixis" {
                n167 = Unbundle By Name(w538) -> ("netCam"=w534:refnum<class "NetworkCamera.lvclass">, "netCamError"=w533:errorcluster)
                n168 = call-dynamic "checkStatus.vi"("error in (no error)"=w533, "stop"=TRUE, "NetworkCamera in"=w534) -> ("error out"=w532:errorcluster, "stopped?"=w530:bool, "NetworkCamera out"=w535:refnum<class "NetworkCamera.lvclass">)  [unwired: 6 in]
                n169 = Bundle By Name(cluster=w538, "netCam"=w535, "netCamError"=w532) -> (w537:refnum<class "AtomChipHWC.lvclass">)
              }
              frame "ProEM" {
                n170 = Unbundle By Name(w548) -> ("netCam"=w544:refnum<class "NetworkCamera.lvclass">, "netCamError"=w539:errorcluster)
                n171 = call-dynamic "checkStatus.vi"("stop"=TRUE, "NetworkCamera in"=w544) -> ("error out"=w541:errorcluster, "stopped?"=w542:bool, "NetworkCamera out"=w545:refnum<class "NetworkCamera.lvclass">)  [unwired: 7 in]
                n172 = Merge Errors(w541, w539) -> (w540:errorcluster)
                n173 = Bundle By Name(cluster=w548, "netCam"=w545, "netCamError"=w540) -> (w547:refnum<class "AtomChipHWC.lvclass">)
              }
            }
            n174 = case shown="True" w264 {
              tunnel: w267 -> [w271 w274]
              tunnel: [w271 w273] -> w266
              tunnel: w265 -> [_ w272]
              frame False {
              }
              frame True {
                n175 = call-dynamic "removedConfiguredDevice.vi"("device"=w272, "HWController in"=w274) -> ("HWController out"=w273:refnum<class "AtomChipHWC.lvclass">)  [unwired: 8 in, 1 out]
              }
            }
          }
          n176 = Search 1D Array(1D array=w248, element=FALSE) -> (index of element=w250:i32)  [unwired: 1 in]
          n177 = Equal?(x=w250, y=-1) -> (x = y?=w247:bool)
        }
      }
      n178 = case shown="False" w9 {
        tunnel: w11 -> [w21 w26]
        tunnel: [w15 w25] -> w8
        tunnel: w10 -> [w20 w24]
        tunnel: [w16 w23] -> w7
        frame True {
          n179 = call "changeStatus.vi"("error in (no error)"=w20, "status"=T1."Stopping", "HWController in"=w21) -> ("error out"=w17:errorcluster, "HWController out"=w18:refnum<class "AtomChipHWC.lvclass">)  [unwired: 7 in]
          n180 = call "removeConfiguredDevices.vi"("error in (no error)"=w17, "HWController in"=w18) -> ("error out"=w16:errorcluster, "HWController out"=w15:refnum<class "AtomChipHWC.lvclass">)  [unwired: 8 in]
        }
        frame False {
          n181 = call "changeStatus.vi"("error in (no error)"=w24, "status"=T1."Running", "HWController in"=w26) -> ("error out"=w23:errorcluster, "HWController out"=w25:refnum<class "AtomChipHWC.lvclass">)  [unwired: 7 in]
        }
      }
    }
    frame Error {
    }
  }
  "error out" <- w3
  "AtomChipHWC out" <- w5
  "stopped" <- w1
